vi "Configure Protect RMS OCP Limit.vi"(7 "Type":enum16{"MIN", "MAX"}(ring), 8 "error in":errorcluster, 9 "Level(A)":dbl min=0.0, 10 "Phase":enum16{"A", "B", "C", "ALL"}(ring), 11 "VISA resource name":refnum<visa-resource-name>) -> (0 "error out":errorcluster, 3 "VISA resource name out":refnum<visa-resource-name>)   [LabVIEW 2020, in "IT-M7700.lvlib"]
doc: "The OCPrms command sets the maximum OCPrms value of a power supply.\n<b>Phase</b>\n0: A\n1: B\n2: C\n3: ALL\n<b>Type</b>\n0: MIN\n1: MAX\n<b>Level(A)</b>\n0-MAX"
uses:
  <instrlib>/IT-M7700/IT-M7700.lvlib
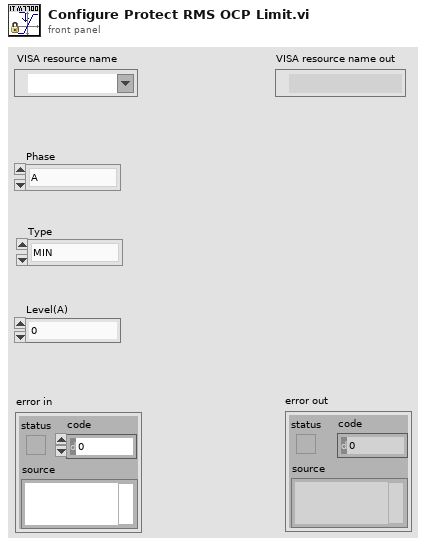
[diagram p1: front panel]
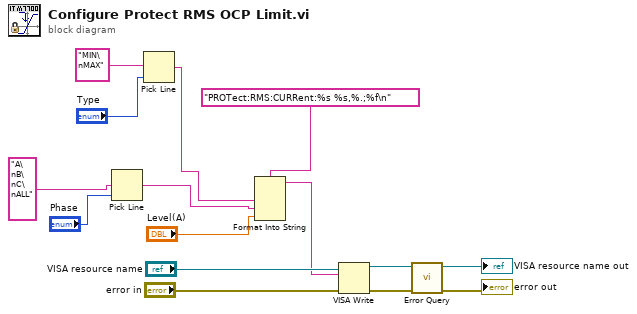
[diagram p0: block diagram]
diagram:
  n1 = Pick Line(multi-line string="A\nB\nC\nALL" ("多行字符串"), line index="Phase") -> (output string=w6:string)  [unwired: 1 in]
  n2 = Pick Line(multi-line string="MIN\nMAX" ("多行字符串"), line index="Type") -> (output string=w2:string)  [unwired: 1 in]
  n3 = Format Into String(format string="PROTect:RMS:CURRent:%s %s,%.;%f\n", w2, w6, "Level(A)") -> (resulting string=w13:string)  [unwired: 2 in, 1 out]
  n4 = VISA Write(VISA resource name="VISA resource name", write buffer=w13, error in (no error)="error in") -> (VISA resource name out=w12:refnum<visa-resource-name>, error out=w11:errorcluster)  [unwired: 1 out]
  n5 = call <instrlib>:"Error Query.vi"("error in"=w11, "VISA resource name"=w12) -> ("error out"=→"error out":errorcluster, "VISA resource name out"=→"VISA resource name out":refnum<visa-resource-name>)  [unwired: 6 in, 2 out]
